vi "svmdense_cross_validation.vi"(8 "error in (no error)":errorcluster, 9 "Nr fold":i32 caption="Nr fold (LOO)", 10 "Parameters":T2, 11 "Problem":T1) -> (0 "error out":errorcluster, 3 "Target":dbl[](array[numeric]) caption="Target (Predicted labels)")   [LabVIEW 2015]
uses:
  LibSVM Sparse/Wrapper API/Controls/svm_parameter.ctl
  LibSVM Sparse/Wrapper API/Controls/svm_type.ctl
  LibSVM Sparse/Wrapper API/Controls/svm_kernel_type.ctl
  Controls/svmdense_problem.ctl
  bin/x64/LabVIEW-libsvm-dense.dll
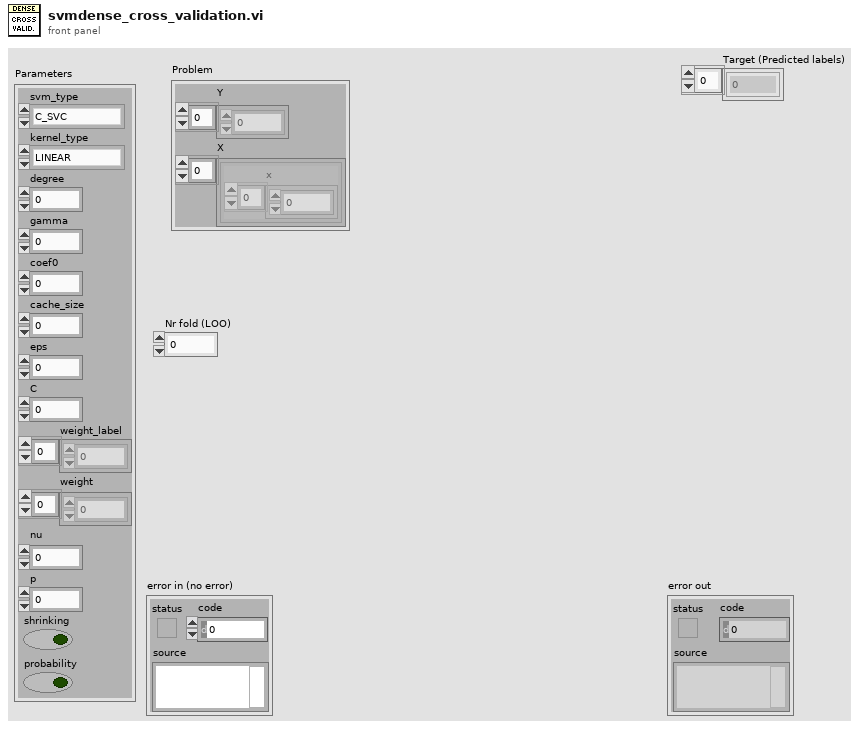
[diagram p1: front panel]
types:
  T1 = typedef "svmdense_problem.ctl" = cluster{"Y":dbl[], "X":cluster{"x":dbl[]}[]}
  T2 = typedef "svm_parameter.ctl" = cluster{"svm_type":T3, "kernel_type":T4, "degree":i32, "gamma":dbl, "coef0":dbl, "cache_size":dbl, "eps":dbl, "C":dbl, "weight_label":i32[], "weight":dbl[], "nu":dbl, "p":dbl, "shrinking":bool, "probability":bool}
  T3 = typedef "svm_type.ctl" = enum32{"C_SVC", "NU_SVC", "ONE_CLASS", "EPSILON_SVR", "NU_SVR"}
  T4 = typedef "svm_kernel_type.ctl" = enum32{"LINEAR", "POLY", "RBF", "SIGMOID", "PRECOMPUTED"}
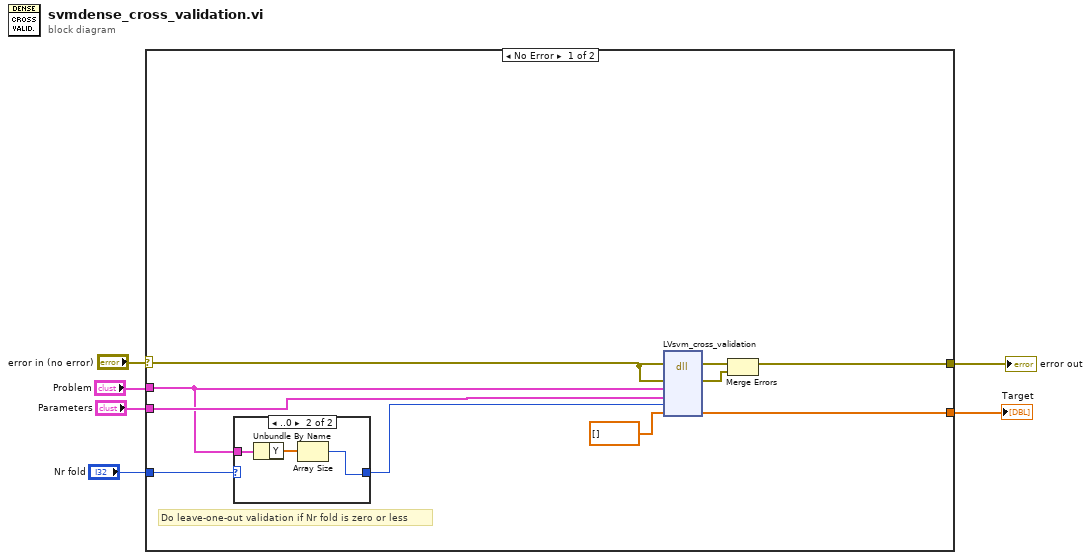
[diagram p0: block diagram]
diagram:
  n1 = case shown="No Error" "error in (no error)" {
    selector: "error in (no error)" -> [w16 w21]
    tunnel: [w15 w21] -> w5
    tunnel: "Nr fold" -> [w12 _]
    tunnel: "Problem" -> [w11 _]
    tunnel: "Parameters" -> [w14 _]
    tunnel: [w13 _] -> w2
    frame No Error {
      # "Do leave-one-out validation if Nr fold is zero or less"
      n2 = case shown="..0" w12 {
        selector: w12 -> [w17 _]
        tunnel: w11 -> [_ w20]
        tunnel: [w17 w18] -> w10
        frame Default {
        }
        frame ..0 {
          n3 = Unbundle By Name(w20) -> ("Y"=w19:dbl[])
          n4 = Array Size(array=w19) -> (size(s)=w18:i32)
        }
      }
      n5 = dll-call lib="C:/dev/LabVIEW-libsvm/LabVIEW/bin/x64/LabVIEW-libsvm-dense.*" fn="LVsvm_cross_validation"(error in=w16, "lvErr"=w16, "prob_in"=w11, "param_in"=w14, "nr_fold"=w10, "target_out"=dbl[] []) -> (error out=w9:errorcluster, "lvErr"=w8:errorcluster, "target_out"=w13:dbl[])  [unwired: 6 in, 1 out]
      n6 = Merge Errors(w9, w8) -> (w15:errorcluster)
    }
    frame Error {
    }
  }
  "error out" <- w5
  "Target" <- w2
